vi "Masking.vi"(8 "error in":errorcluster, 10 "Number":u64, 11 "Mask in":u64) -> (0 "error out":errorcluster, 2 "x .and. y?":u8, 3 "Mask Data":u32)   [LabVIEW 2023, in "HardwareAbstractionLayer_LVOOP.lvlib" / "Report.lvclass"]
uses:
  Report.lvclass
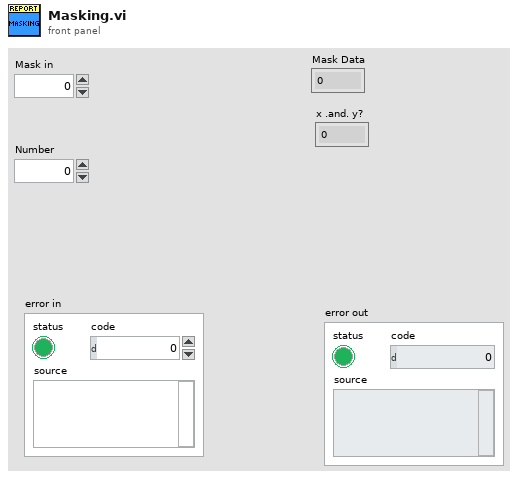
[diagram p1: front panel]
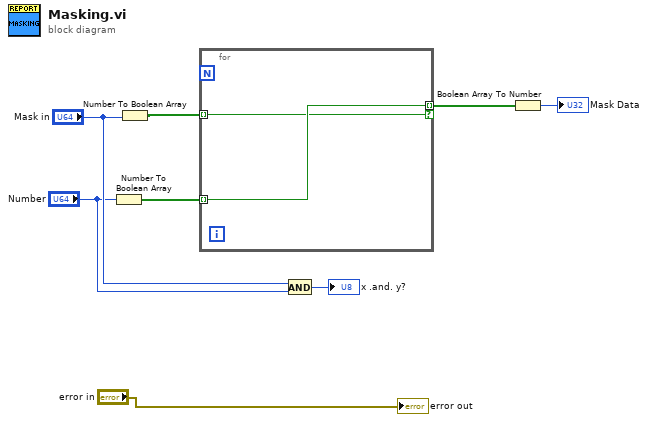
[diagram p0: block diagram]
diagram:
  n1 = Number To Boolean Array(number="Number") -> (Boolean array=w7:bool[])
  n2 = Number To Boolean Array(number="Mask in") -> (Boolean array=w8:bool[])
  n3 = for {
    tunnel: w8 -> [w9] mode=indexing
    tunnel: w7 -> [w10] mode=indexing
    tunnel: [w10] -> w6 mode=indexing if=w9
  }
  n4 = And(x="Mask in", y="Number") -> (x .and. y?=→"x .and. y?":u64)
  n5 = Boolean Array To Number(Boolean array=w6) -> (number=→"Mask Data":u32)
  "error out" <- "error in"
